vi "Write Gains.vi"(8 "error in (no error)":errorcluster, 10 "Gains":cluster{"Red":dbl, "Blue0":dbl, "Blue1":dbl}, 11 "Change Laser Gain CMD in":refnum<class "Change Laser Gain CMD.lvclass">) -> (0 "error out":errorcluster, 3 "Change Laser Gain CMD out":refnum<class "Change Laser Gain CMD.lvclass">)   [LabVIEW 2014, in "eCRDS Library.lvlib" / "Change Laser Gain CMD.lvclass"]
uses:
  Change Laser Gain CMD.lvclass
  Change Laser Gain CMD.lvclass/Change Laser Gain CMD.ctl
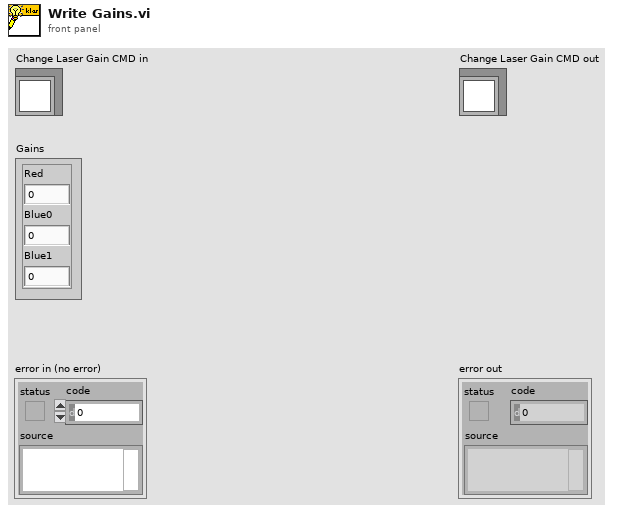
[diagram p1: front panel]
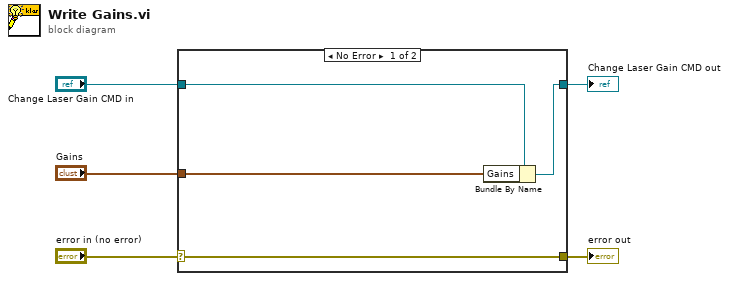
[diagram p0: block diagram]
diagram:
  n1 = case shown="No Error" "error in (no error)" {
    selector: "error in (no error)" -> [w9 w10]
    tunnel: [w9 w10] -> w4
    tunnel: [w7 w11] -> w2
    tunnel: "Change Laser Gain CMD in" -> [w8 w11]
    tunnel: "Gains" -> [w6 _]
    frame No Error {
      n2 = Bundle By Name(cluster=w8, "Gains"=w6) -> (w7:refnum<class "Change Laser Gain CMD.lvclass">)
    }
    frame Error {
    }
  }
  "error out" <- w4
  "Change Laser Gain CMD out" <- w2
